vi "ep_Symmetrical To Unbalance.vi"(0 "symmetrical components":dbl[](array[numeric]), 11 "error in (no error)":errorcluster) -> (4 "unbalance":dbl[](array[numeric]), 15 "error out":errorcluster)   [LabVIEW 2014, in "NI_EP_Power Quality.lvlib"]
uses:
  <vilib>/addons/Electrical Power/PQ/NI_EP_Power Quality.lvlib
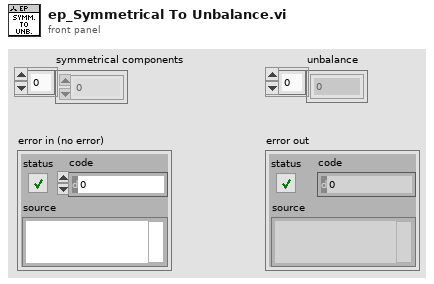
[diagram p1: front panel]
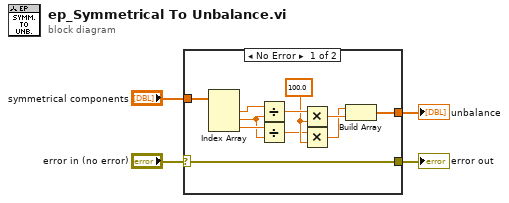
[diagram p0: block diagram]
diagram:
  n1 = case shown="No Error" "error in (no error)" {
    selector: "error in (no error)" -> [w5 w16]
    tunnel: "symmetrical components" -> [w8 _]
    tunnel: [w7 _] -> w3
    tunnel: [w5 w16] -> w1
    frame No Error {
      w11 = 100.0 ("y")
      n2 = Index Array(array=w8) -> (element #1=w14:dbl, element #2=w13:dbl, element #3=w15:dbl)  [unwired: 3 in]
      n3 = Divide(x=w14, y=w13) -> (x/y=w12:dbl)
      n4 = Divide(x=w15, y=w13) -> (x/y=w6:dbl)
      n5 = Multiply(x=w12, y=w11) -> (x*y=w10:dbl)
      n6 = Multiply(x=w6, y=w11) -> (x*y=w9:dbl)
      n7 = Build Array(w9, w10) -> (w7:dbl[])
    }
    frame Error {
    }
  }
  "unbalance" <- w3
  "error out" <- w1
